vi "ampl_phase.vi"(3 "error in":errorcluster, 5 "adress string":string) -> (0 "error out":errorcluster, 1 "amplitude":dbl, 2 "phase shi ft":dbl)   [LabVIEW 2010]
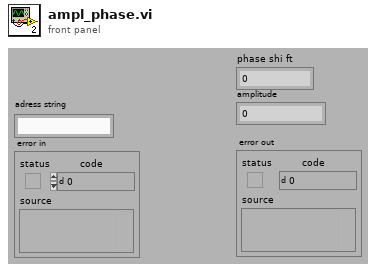
[diagram p1: front panel]
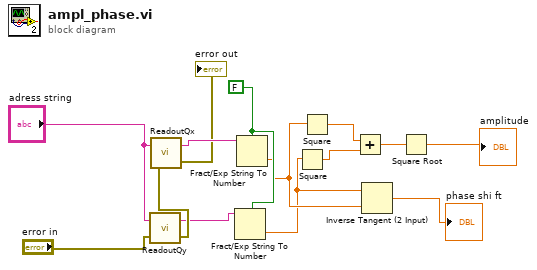
[diagram p0: block diagram]
diagram:
  w12 = FALSE
  n1 = call "ReadoutQy.vi"("error in"="error in", "address string"="adress string") -> ("error out"=w14:errorcluster, "String"=w11:string)
  n2 = call "ReadoutQx.vi"("error in"=w14, "address string"="adress string") -> ("error out"=→"error out":errorcluster, "String"=w13:string)
  n3 = Fract/Exp String To Number(use system decimal point (T)=w12, string=w11) -> (number=w2:dbl)  [unwired: 2 in, 1 out]
  n4 = Fract/Exp String To Number(use system decimal point (T)=w12, string=w13) -> (number=w3:dbl)  [unwired: 2 in, 1 out]
  n5 = Square(x=w2) -> (x^2=w9:dbl)
  n6 = Square(x=w3) -> (x^2=w10:dbl)
  n7 = Add(x=w10, y=w9) -> (x+y=w8:dbl)
  n8 = Inverse Tangent (2 Input)(1:w3, 2:w2) -> (0:→"phase shi ft":dbl)
  n9 = Square Root(x=w8) -> (sqrt(x)=→"amplitude":dbl)
